vi "RT_stage_control_rev8_loadverification.vi"() -> ()   [LabVIEW 2019]
uses:
  StageControl.ctl
  RasterControl.ctl
  ForceControl.ctl
  <vilib>/Platform/TimedLoop/XDataNode/timing_clust.ctl
  <vilib>/Platform/TimedLoop/XDataNode/nitl_modes.ctl
  <vilib>/Platform/TimedLoop/XDataNode/wakeup.ctl
  <vilib>/FPGAPlugInAG/myRIO-1900/niLvFpga_Open_myRIO-1900.vi
  <vilib>/rvi/interface/common/dynamic/niFpgaDynamicAddResources.vi
  <vilib>/Utility/error.llb/Error Cluster From Error Code.vi
  <vilib>/rvi/errors/niLvFpgaAdjustHostInterfaceError.vi
  <vilib>/FPGAPlugInAG/Dynamic/niLvFpga_Close_Dynamic.vi
  <vilib>/rvi/interface/nirviOpenFPGA/nirviOpenFPGA.xnode
  FPGA Bitfiles/studentchallenge_FPGATarget_FPGARADCWDAC3_YedoVmsa1Hg.lvbitx
  FPGA_2R_ADC_W_DAC.vi
  <vilib>/Platform/TimedLoop/XDataNode/XDataNode.xnode
  <vilib>/rvi/interface/nirviReadWriteControl/nirviReadWriteControl.xnode
  <vilib>/rvi/interface/nirviCloseFPGA/nirviCloseFPGA.xnode
  <vilib>/Platform/TimedLoop/XDataNode/XDNodeRunTimeDep.lvlib
  NiFpgaLv.dll
  <vilib>/rvi/interface/Simulation/niFpgaSimulationCallBeginRW.vi
panel:
  out "load cell out":dbl(graph)
  out "Force Loop":T1
  out "Force Control Late":i16
  in  "Y Manual [mm]":dbl format="%.4f"
  in  "X Manual [mm]":dbl format="%.4f"
  in  "Zero Cap":bool
  in  "Zero Y":bool
  in  "Zero X":bool
  in  "Des Force [N]":dbl=0.3 format="%.3f"
  in  "Return Speed":dbl=5.0 format="%#_13g"
  in  "Step Size [mm]":dbl=0.02 format="%.3f"
  in  "Width [mm]":dbl=3.0 format="%.3f"
  in  "Velocity [mm/s]":dbl=0.1 format="%.3f"
  in  "Stroke [mm]":dbl=3.0 format="%.3f"
  out "Current [A]":dbl=-0.00198361231060317 format="%.4f"
  out "Cap Probe [mm]":dbl=0.43435006179715263 format="%.4f"
  out "X Position [mm]":dbl format="%.4f"
  out "Y Position [mm]":dbl=0.0003125 format="%.4f"
  out "Stage Motion Late":i16
  in  "Start":bool
  in  "Operation":T2=enum."Raster"
  out "Raster Loop":T3
  out "Outer Loop":T2
  in  "stop":bool
  out "settle start":u32
  out "stroke finished":bool=TRUE
  out "ToolDownStart":bool
  out "Tool Up Finished":bool
  out "Tool Down Finished":bool
  out "FPGA Ref":refnum<k20>
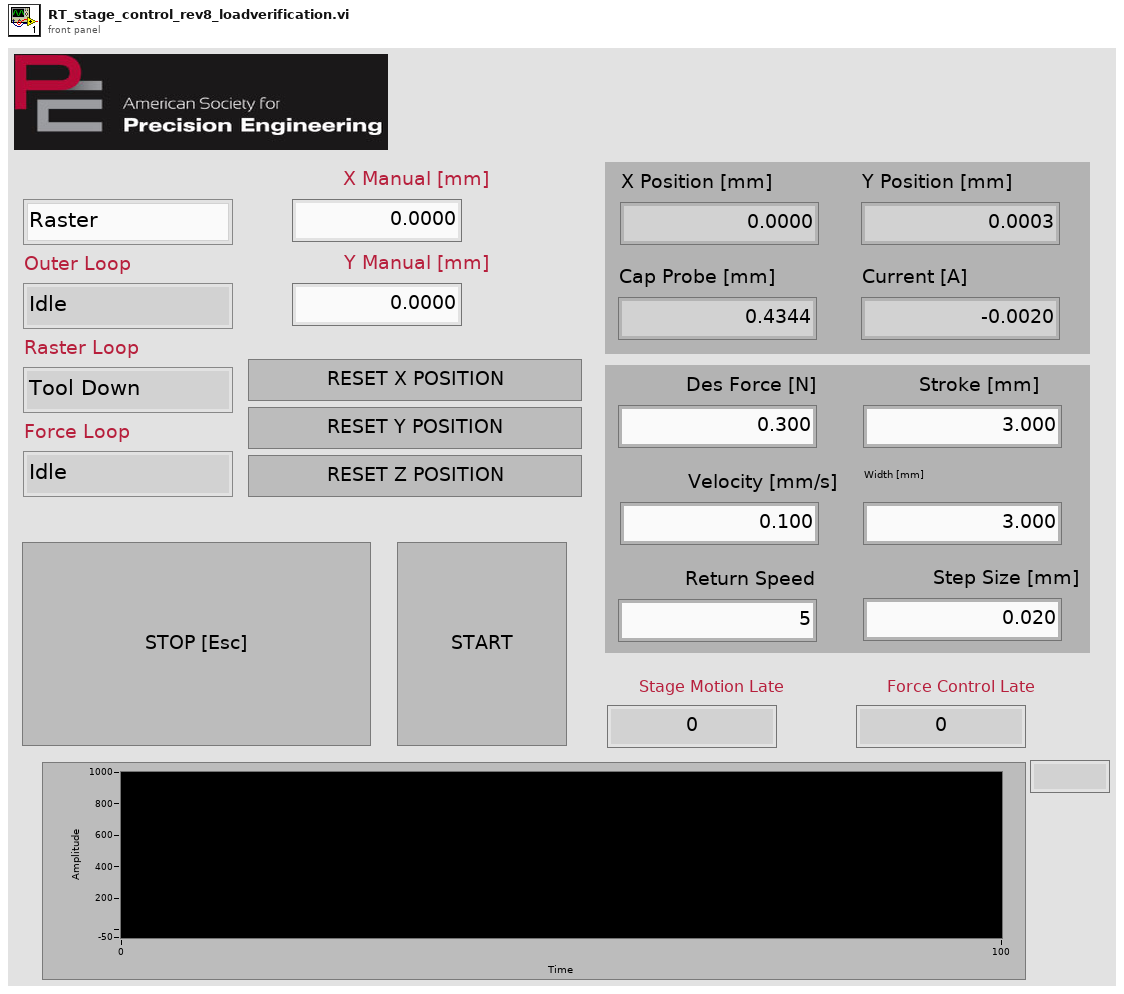
[diagram p1: front panel]
types:
  T1 = typedef "ForceControl.ctl" = enum16{"Idle", "Tool Down", "Force Control", "Tool Up"}
  T2 = typedef "StageControl.ctl" = enum16{"Idle", "Raster", "Home X", "Home Y"}
  T3 = typedef "RasterControl.ctl" = enum16{"Tool Down", "Stroke", "Tool Up", "Return & Step", "Settle", "Return to Zero"}
  T4 = cluster{"Encoder A":i32, "Encoder B":i32, "X Desired [mm]":dbl, "X Position [mm]":dbl, "Y Desired [mm]":dbl, "Y Position [mm]":dbl}
  T5 = typedef "XDNodeRunTimeDep.lvlib/timing_clust.ctl" = cluster{"Expected End [f-1]":u64, "Actual End [f-1]":u64, "Finished Late? [f-1]":bool, "Expected End [i-1]":u64, "Actual End [i-1]":u64, "Finished Late? [i-1]":bool, "Expected Start [i]":u64, "Actual Start [i]":u64, "Expected Start [f]":u64, "Actual Start [f]":u64, "Source Name":string, "Structure Name":string, "Period":i64, "Deadline":i64, "Offset":i64, "Start":i64, "Priority":i32, "Timeout":i32, "Mode":T6, "Wakeup Reason":T7, "Error":errorcluster, "Source Type":string, "Secondary Source Type":string, "Global End Time":u64, "Global Start Time":u64, "Frame Duration":u64, "Iteration Duration":u64, "Assigned CPU":i32, "I/O Scan Engine Mode":u32}
  T6 = typedef "XDNodeRunTimeDep.lvlib/nitl_modes.ctl" = enum32{"No Change", "Process missed periods, maintain original phase", "Discard missed periods, maintain original phase", "Process missed periods, ignore original phase", "Discard missed periods, ignore original phase"}
  T7 = typedef "XDNodeRunTimeDep.lvlib/wakeup.ctl" = enum32{"Normal", "Aborted", "Asynchronous wakeup", "Timing source error", "Timed loop error", "Timeout"}
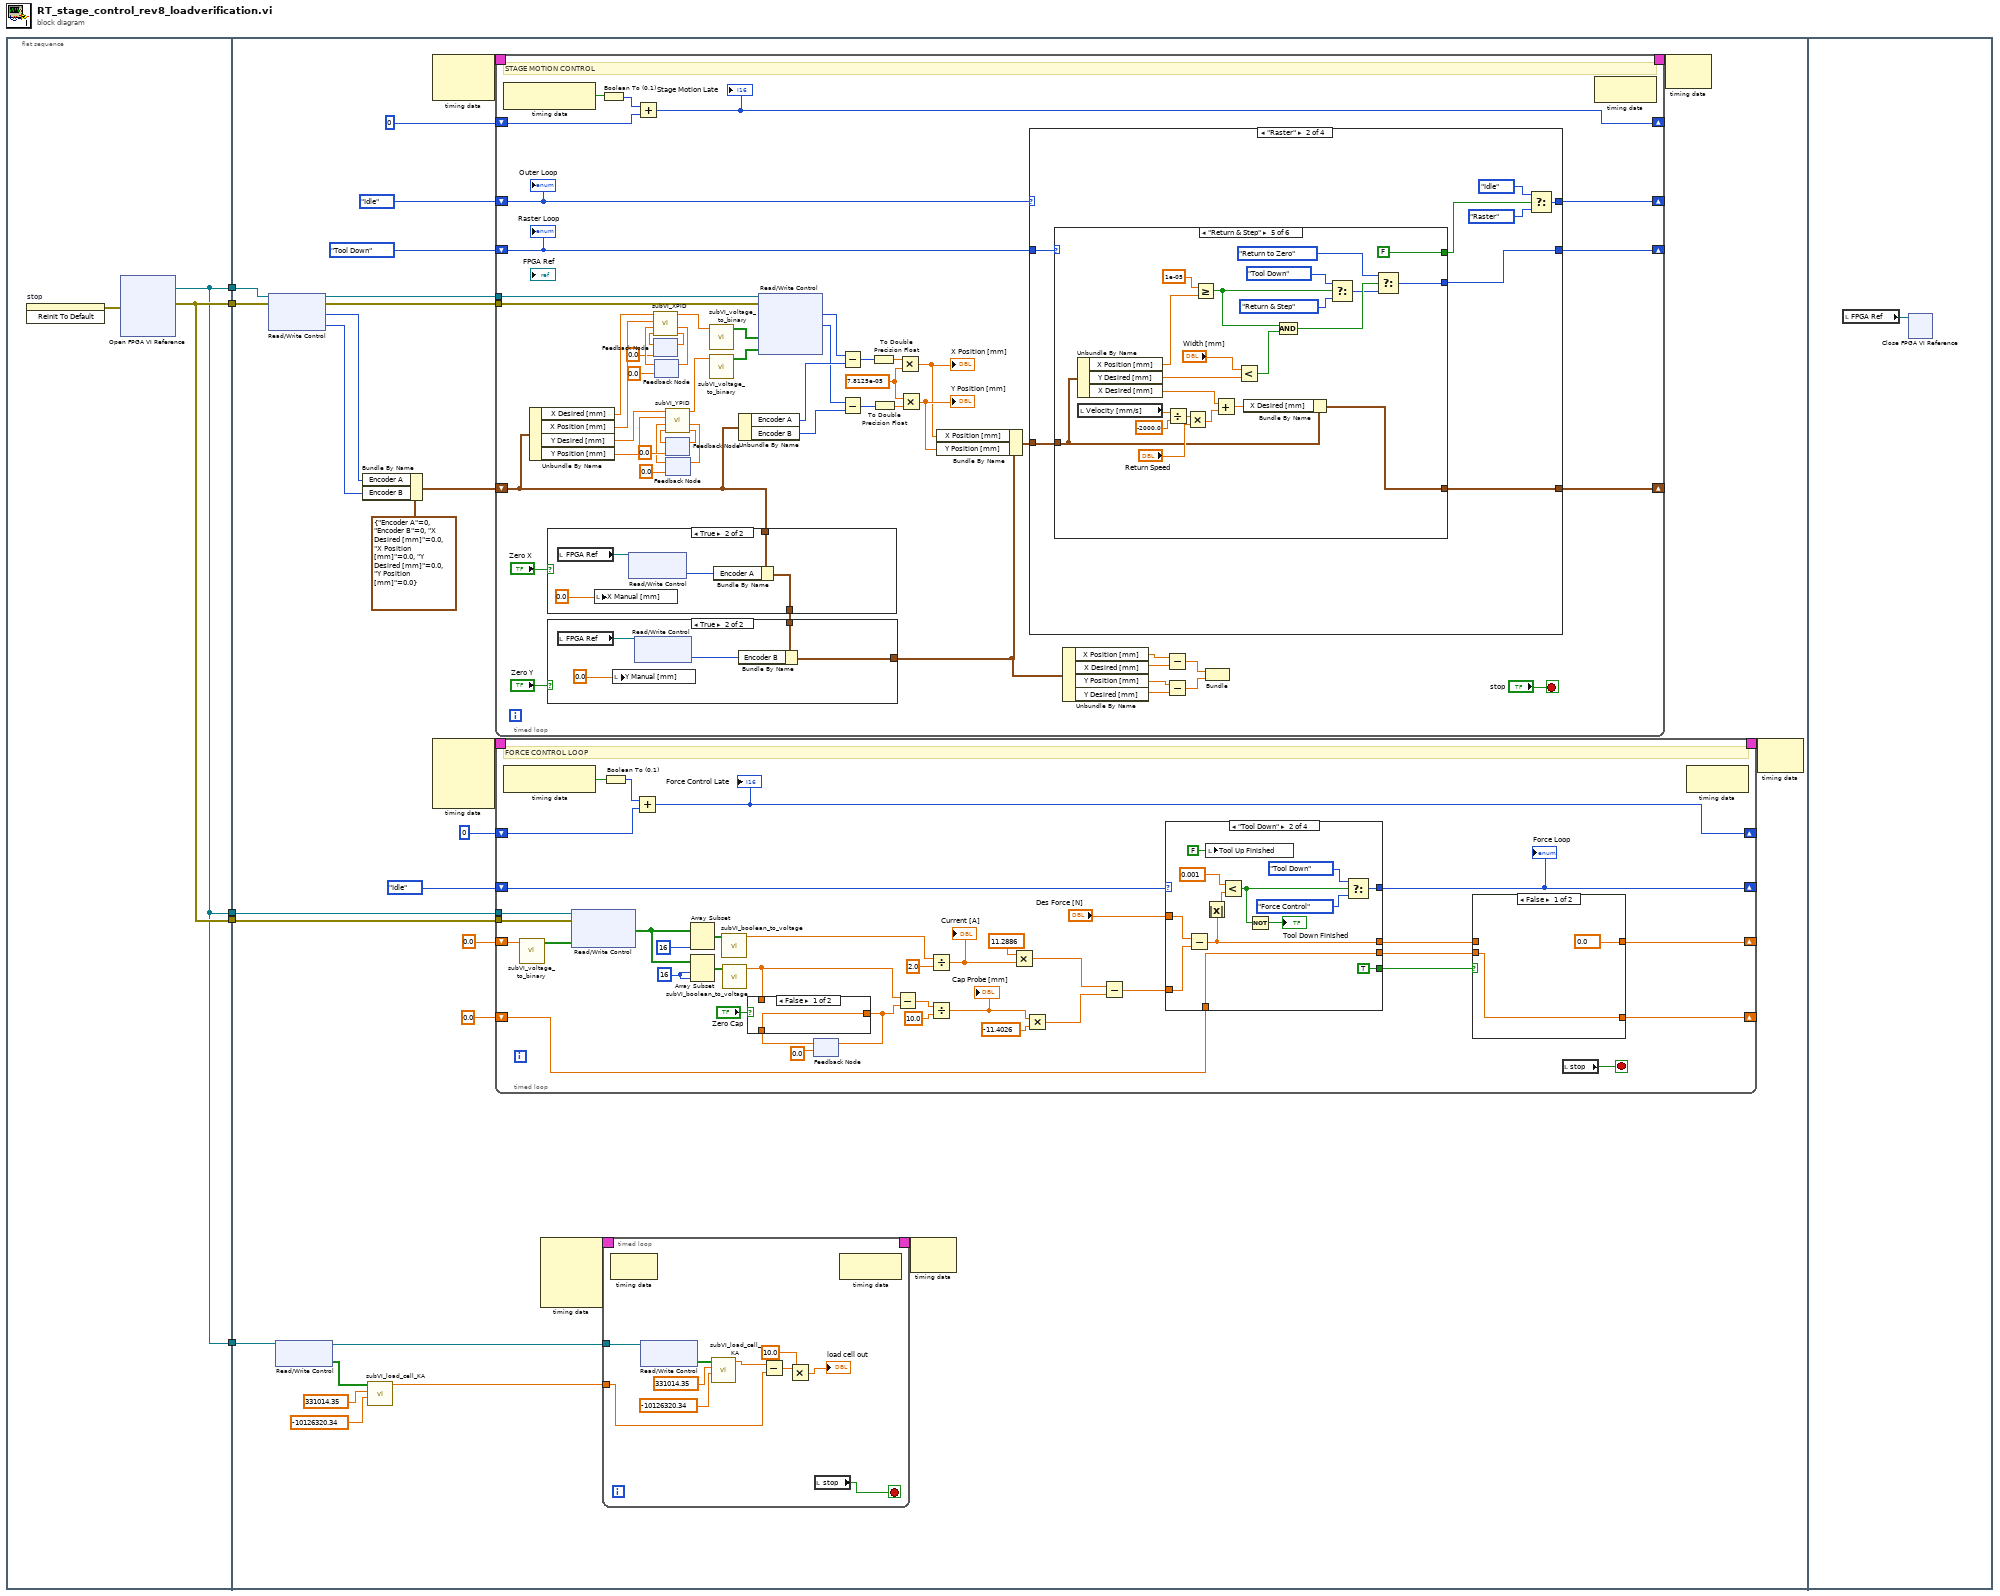
[diagram p0: block diagram]
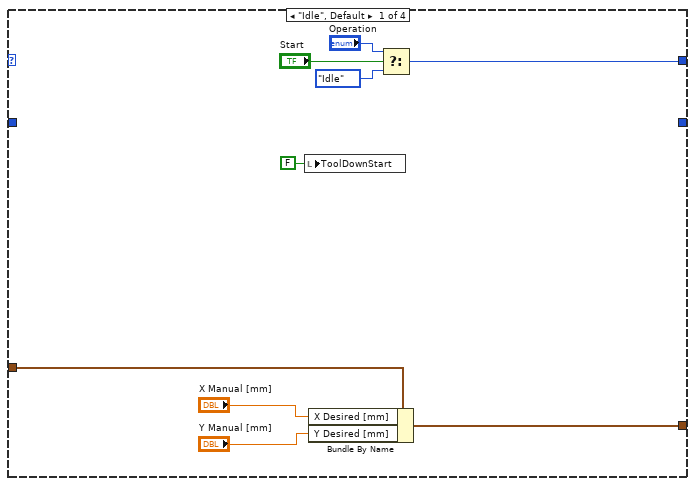
[diagram p2: hidden frame]
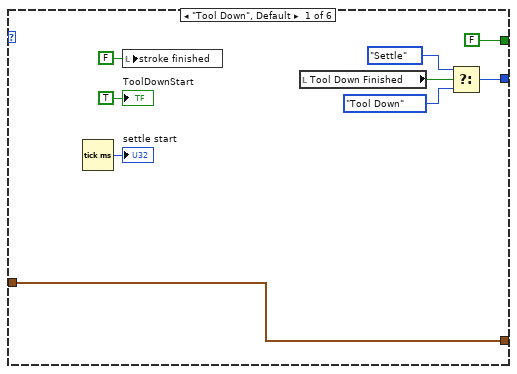
[diagram p3: hidden frame]
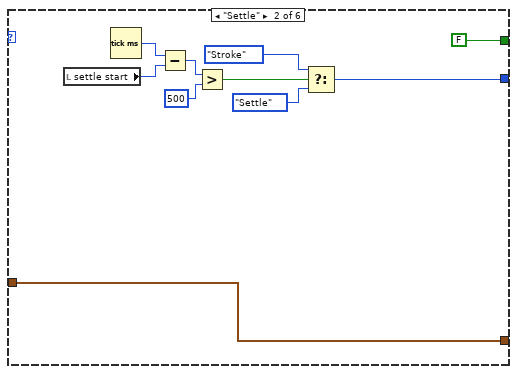
[diagram p4: hidden frame]
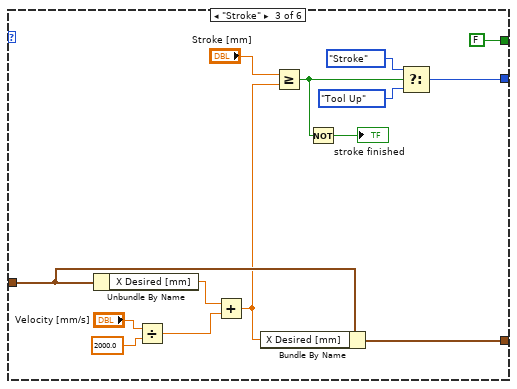
[diagram p5: hidden frame]
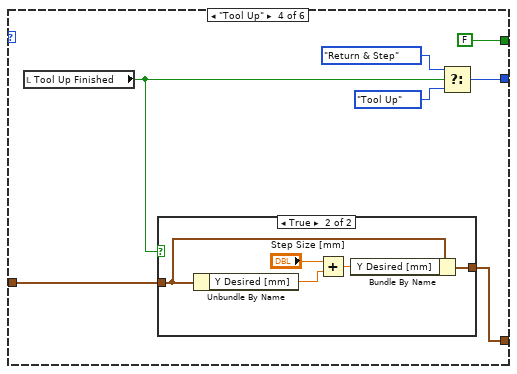
[diagram p6: hidden frame]
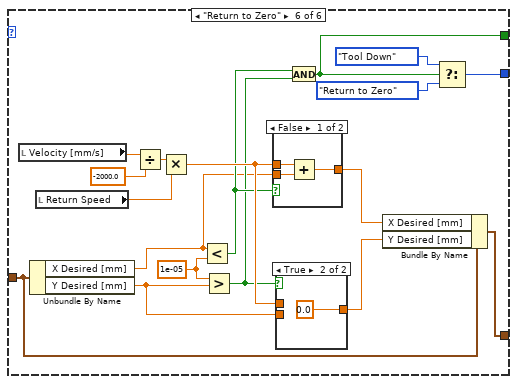
[diagram p8: hidden frame]
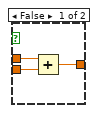
[diagram p9: hidden frame]
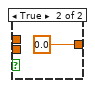
[diagram p10: hidden frame]
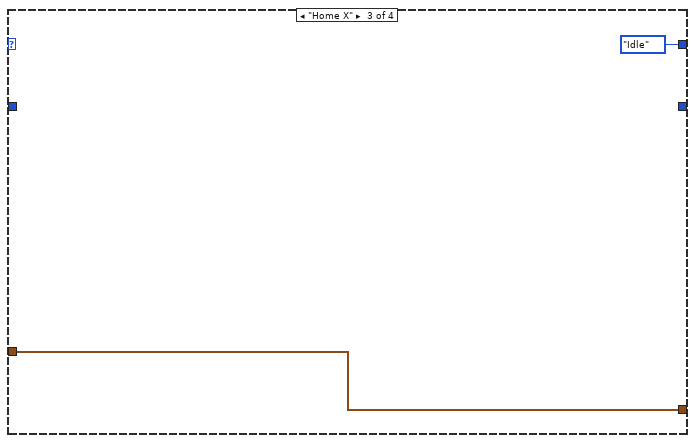
[diagram p11: hidden frame]
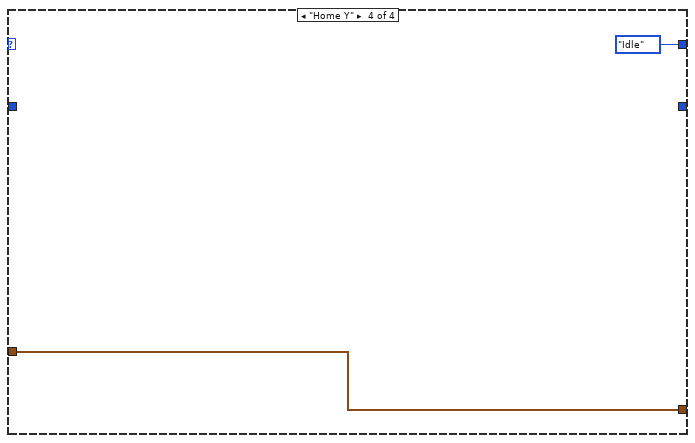
[diagram p12: hidden frame]
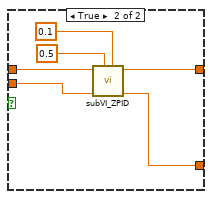
[diagram p15: hidden frame]
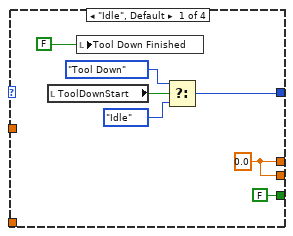
[diagram p17: hidden frame]
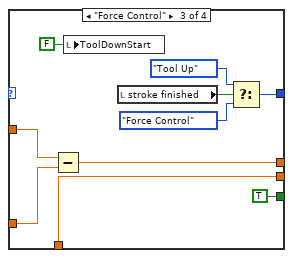
[diagram p18: hidden frame]
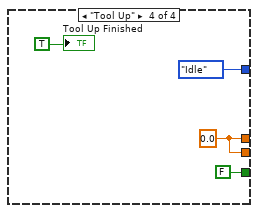
[diagram p19: hidden frame]
diagram:
  n1 = flat-sequence {
    tunnel: [w7] -> w5
    tunnel: [w6] -> w4
    tunnel: [w6] -> w3
    tunnel: [w7] -> w2
    tunnel: [w6] -> w1
    tunnel: w5 -> [w28]
    tunnel: w4 -> [w26]
    tunnel: w3 -> [w15]
    tunnel: w2 -> [w25]
    tunnel: w1 -> [w14]
    frame #0 {
      n2 = invoke on="stop" class="Bool (strict)" method="Reinit To Default"() -> (error out=w8:errorcluster)  [unwired: 3 in, 2 out]
      n3 = xnode "Open FPGA VI Reference"("error in"=w8) -> ("FPGA VI Reference Out"=w6:refnum<k20>, "error out"=w7:errorcluster)  [unwired: 1 in]
    }
    frame #1 {
      n4 = xnode "Read/Write Control"("FPGA VI Reference In"=w26, "error in"=w28) -> ("FPGA VI Reference Out"=w33:refnum<k20>, "error out"=w32:errorcluster, "Encoder A"=w21:i32, "Encoder B"=w22:i32)
      n5 = xnode "Read/Write Control"("FPGA VI Reference In"=w14) -> ("FPGA VI Reference Out"=w13:refnum<k20>, "Data array"=w12:bool[])  [unwired: 1 in, 1 out]
      n6 = Bundle By Name(cluster=T4 {"Encoder A"=0, "Encoder B"=0, "X Desired [mm]"=0.0, "X Position [mm]"=0.0, "Y Desired [mm]"=0.0, "Y Position [mm]"=0.0}, "Encoder A"=w21, "Encoder B"=w22) -> (w23:T4)
      n7 = call "subVI_load_cell_KA.vi"("offset"=-10126320.34, "scale"=331014.35, "DATA ARRAY IN"=w12) -> ("LOAD OUT"=w9:dbl)  [unwired: 8 in]
      n8 = node-c288() -> (w37:T5)  [unwired: 2 in]
      n9 = node-c288() -> (w35:T5)  [unwired: 4 in]
      n10 = timed-loop {
        timing: w37 -> [_]
        timing-out: [_] -> w36
        tunnel: w33 -> [w52]
        tunnel: w32 -> [w105]
        shift-right: [w99] -> _
        shift-left: StageControl."Idle" ("Enum 2") -> [w98]
        shift-right: [w96] -> _
        shift-left: RasterControl."Tool Down" -> [w97]
        shift-right: [w90] -> _
        shift-left: i16 0 -> [w91]
        shift-right: [w72] -> _
        shift-left: w23 -> [w67]
        stop <- "stop" stop-if-true
        w100 = 7.8125e-05 ("y")
        # "STAGE MOTION CONTROL"
        n11 = node-c288() -> (w93:bool)  [unwired: 1 in]
        n12 = Unbundle By Name(w67) -> ("X Desired [mm]"=w71:dbl, "X Position [mm]"=w70:dbl, "Y Desired [mm]"=w69:dbl, "Y Position [mm]"=w68:dbl)
        n13 = case shown="True" "Zero X" {
          tunnel: [w231 w233] -> w73
          tunnel: w67 -> [w231 w232]
          frame False {
          }
          frame True {
            n14 = local read "FPGA Ref"() -> (w235:refnum<k20>)
            n15 = local write "X Manual [mm]"(0.0 ("X Relative Position [mm]")) -> ()
            n16 = xnode "Read/Write Control"("FPGA VI Reference In"=w235) -> ("Encoder A"=w234:i32)  [unwired: 1 in, 2 out]
            n17 = Bundle By Name(cluster=w232, "Encoder A"=w234) -> (w233:T4)
          }
        }
        n18 = case shown="True" "Zero Y" {
          tunnel: w73 -> [w225 w229]
          tunnel: [w225 w226] -> w53
          frame False {
          }
          frame True {
            n19 = local read "FPGA Ref"() -> (w230:refnum<k20>)
            n20 = local write "Y Manual [mm]"(0.0 ("Y Relative Position [mm]")) -> ()
            n21 = xnode "Read/Write Control"("FPGA VI Reference In"=w230) -> ("Encoder B"=w228:i32)  [unwired: 1 in, 2 out]
            n22 = Bundle By Name(cluster=w229, "Encoder B"=w228) -> (w226:T4)
          }
        }
        n23 = Boolean To (0,1)(Boolean=w93) -> (0, 1=w92:i16)
        n24 = Add(x=w92, y=w91) -> (x+y=w90:i16)
        "Stage Motion Late" <- w90
        n25 = feedback #1(0.0 ("Cumulative Error Out")) -> (w85:dbl)
        n26 = feedback #2(0.0 ("Error")) -> (w84:dbl)
        n27 = call "subVI_XPID.vi"("Cumulative Error In"=w85, "Previous Error"=w84, "Encoder Position [mm]"=w70, "Desired Position [mm]"=w71) -> ("Cumulative Error Out"=w87:dbl, "Error"=w86:dbl, "Control Signal [V]"=w75:dbl)  [unwired: 5 in]
        n28 = feedback-in #1(w87) -> ()
        n29 = feedback-in #2(w86) -> ()
        n30 = feedback #3(0.0 ("Cumulative Error Out")) -> (w78:dbl)
        n31 = feedback #4(0.0 ("Error")) -> (w79:dbl)
        n32 = call "subVI_YPID.vi"("Cumulative Error In"=w78, "Previous Error"=w79, "Encoder Position [mm]"=w68, "Desired Position [mm]"=w69) -> ("Cumulative Error Out"=w76:dbl, "Error"=w77:dbl, "Control Signal [V]"=w74:dbl)  [unwired: 5 in]
        n33 = feedback-in #3(w76) -> ()
        n34 = feedback-in #4(w77) -> ()
        n35 = call "subVI_voltage_to_binary.vi"("voltage"=w75) -> ("binary"=w89:bool[])  [unwired: 10 in]
        n36 = call "subVI_voltage_to_binary.vi"("voltage"=w74) -> ("binary"=w88:bool[])  [unwired: 10 in]
        n37 = Unbundle By Name(w67) -> ("Encoder A"=w66:i32, "Encoder B"=w65:i32)
        n38 = xnode "Read/Write Control"("FPGA VI Reference In"=w52, "error in"=w105, "DAC 1 write"=w89, "DAC 2 write"=w88) -> ("Encoder A"=w64:i32, "Encoder B"=w63:i32)  [unwired: 2 out]
        n39 = Subtract(x=w64, y=w66) -> (x-y=w103:i32)
        n40 = Subtract(x=w63, y=w65) -> (x-y=w102:i32)
        n41 = To Double Precision Float(number=w103) -> (double precision float=w104:dbl)
        n42 = To Double Precision Float(number=w102) -> (double precision float=w101:dbl)
        n43 = Multiply(x=w104, y=w100) -> (x*y=w60:dbl)
        "X Position [mm]" <- w60
        n44 = Multiply(x=w100, y=w101) -> (x*y=w61:dbl)
        "Y Position [mm]" <- w61
        n45 = Bundle By Name(cluster=w53, "X Position [mm]"=w60, "Y Position [mm]"=w61) -> (w62:T4)
        n46 = case shown="\"Raster\"" w98 {
          tunnel: [w118 w125 StageControl."Idle" ("Enum 2") StageControl."Idle" ("Enum 2")] -> w99
          tunnel: w97 -> [_ w126 _ _]
          tunnel: [_ w121 _ _] -> w96
          tunnel: w62 -> [w110 w120 w221 w223]
          tunnel: [w111 w119 w221 w223] -> w72
          frame "Idle", Default {
            n47 = local write "ToolDownStart"(FALSE ("ToolDownStart")) -> ()
            n48 = Bundle By Name(cluster=w110, "X Desired [mm]"="X Manual [mm]", "Y Desired [mm]"="Y Manual [mm]") -> (w111:T4)
            n49 = Select(t="Operation", s="Start", f=StageControl."Idle" ("Enum 2")) -> (s? t:f=w118:T2)
          }
          frame "Raster" {
            n50 = case shown="\"Return & Step\"" w126 {
              tunnel: [FALSE FALSE FALSE FALSE FALSE w207] -> w122
              tunnel: [w134 w144 w156 w161 w177 w209] -> w121
              tunnel: [w128 w136 w153 w164 w181 w200] -> w119
              tunnel: w120 -> [w128 w136 w150 w160 w173 w197]
              frame "Tool Down", Default {
                n51 = Tick Count (ms)() -> (millisecond timer value=→"settle start":u32)
                n52 = local write "stroke finished"(FALSE ("stroke finished")) -> ()
                n53 = local read "Tool Down Finished"() -> (w131:bool)
                n54 = Select(t=RasterControl."Settle", s=w131, f=RasterControl."Tool Down") -> (s? t:f=w134:T3)
                "ToolDownStart" <- TRUE
              }
              frame "Settle" {
                n55 = local read "settle start"() -> (w137:u32)
                n56 = Tick Count (ms)() -> (millisecond timer value=w142:u32)
                n57 = Subtract(x=w142, y=w137) -> (x-y=w141:u32)
                n58 = Greater?(x=w141, y=u32 500) -> (0:w138:bool)
                n59 = Select(t=RasterControl."Stroke", s=w138, f=RasterControl."Settle") -> (s? t:f=w144:T3)
              }
              frame "Stroke" {
                n60 = Unbundle By Name(w150) -> ("X Desired [mm]"=w149:dbl)
                n61 = Divide(x="Velocity [mm/s]", y=2000.0) -> (x/y=w151:dbl)
                n62 = Add(x=w149, y=w151) -> (x+y=w148:dbl)
                n63 = Bundle By Name(cluster=w150, "X Desired [mm]"=w148) -> (w153:T4)
                n64 = Greater Or Equal?(x="Stroke [mm]", y=w148) -> (x >= y?=w147:bool)
                n65 = Not(x=w147) -> (.not. x?=→"stroke finished":bool)
                n66 = Select(t=RasterControl."Stroke", s=w147, f=RasterControl."Tool Up") -> (s? t:f=w156:T3)
              }
              frame "Tool Up" {
                n67 = local read "Tool Up Finished"() -> (w163:bool)
                n68 = case shown="True" w163 {
                  tunnel: [w167 w171] -> w164
                  tunnel: w160 -> [w167 w168]
                  frame False {
                  }
                  frame True {
                    n69 = Unbundle By Name(w168) -> ("Y Desired [mm]"=w169:dbl)
                    n70 = Add(x="Step Size [mm]", y=w169) -> (x+y=w172:dbl)
                    n71 = Bundle By Name(cluster=w168, "Y Desired [mm]"=w172) -> (w171:T4)
                  }
                }
                n72 = Select(t=RasterControl."Return & Step", s=w163, f=RasterControl."Tool Up") -> (s? t:f=w161:T3)
              }
              frame "Return & Step" {
                n73 = Unbundle By Name(w173) -> ("X Position [mm]"=w175:dbl, "Y Desired [mm]"=w174:dbl, "X Desired [mm]"=w176:dbl)
                n74 = local read "Velocity [mm/s]"() -> (w192:dbl)
                n75 = Divide(x=w192, y=-2000.0) -> (x/y=w190:dbl)
                n76 = Multiply(x=w190, y="Return Speed") -> (x*y=w182:dbl)
                n77 = Greater Or Equal?(x=1e-05 ("y"), y=w175) -> (x >= y?=w184:bool)
                n78 = Add(x=w176, y=w182) -> (x+y=w183:dbl)
                n79 = Less?(x="Width [mm]", y=w174) -> (x < y?=w178:bool)
                n80 = Bundle By Name(cluster=w173, "X Desired [mm]"=w183) -> (w181:T4)
                n81 = And(x=w184, y=w178) -> (x .and. y?=w187:bool)
                n82 = Select(t=RasterControl."Tool Down", s=w184, f=RasterControl."Return & Step") -> (s? t:f=w186:T3)
                n83 = Select(t=RasterControl."Return to Zero", s=w187, f=w186) -> (s? t:f=w177:T3)
              }
              frame "Return to Zero" {
                w204 = 1e-05 ("y")
                n84 = local read "Velocity [mm/s]"() -> (w212:dbl)
                n85 = Unbundle By Name(w197) -> ("X Desired [mm]"=w196:dbl, "Y Desired [mm]"=w195:dbl)
                n86 = local read "Return Speed"() -> (w205:dbl)
                n87 = Divide(x=w212, y=-2000.0) -> (x/y=w210:dbl)
                n88 = Multiply(x=w210, y=w205) -> (x*y=w203:dbl)
                n89 = Less?(x=w196, y=w204) -> (x < y?=w199:bool)
                n90 = Greater?(x=w204, y=w195) -> (0:w198:bool)
                n91 = case shown="False" w199 {
                  tunnel: w203 -> [w219 _]
                  tunnel: [w218 0.0] -> w202
                  tunnel: w196 -> [w217 _]
                  frame False {
                    n92 = Add(x=w219, y=w217) -> (x+y=w218:dbl)
                  }
                  frame True {
                  }
                }
                n93 = case shown="True" w198 {
                  tunnel: w203 -> [w215 _]
                  tunnel: [w214 0.0] -> w201
                  tunnel: w195 -> [w213 _]
                  frame False {
                    n94 = Add(x=w215, y=w213) -> (x+y=w214:dbl)
                  }
                  frame True {
                  }
                }
                n95 = And(x=w199, y=w198) -> (x .and. y?=w207:bool)
                n96 = Bundle By Name(cluster=w197, "X Desired [mm]"=w202, "Y Desired [mm]"=w201) -> (w200:T4)
                n97 = Select(t=RasterControl."Tool Down", s=w207, f=RasterControl."Return to Zero") -> (s? t:f=w209:T3)
              }
            }
            n98 = Select(t=StageControl."Idle" ("Enum 2"), s=w122, f=StageControl."Raster" ("Enum 2")) -> (s? t:f=w125:T2)
          }
          frame "Home X" {
          }
          frame "Home Y" {
          }
        }
        n99 = Unbundle By Name(w53) -> ("X Position [mm]"=w56:dbl, "X Desired [mm]"=w57:dbl, "Y Position [mm]"=w58:dbl, "Y Desired [mm]"=w59:dbl)
        n100 = Subtract(x=w56, y=w57) -> (x-y=w55:dbl)
        n101 = Subtract(x=w58, y=w59) -> (x-y=w54:dbl)
        n102 = Bundle(w55, w54) -> ()  [unwired: 1 in, 1 out]
        n103 = node-c288() -> ()  [unwired: 1 in, 1 out]
        "Outer Loop" <- w98
        "Raster Loop" <- w97
      }
      n104 = timed-loop {
        timing: w35 -> [_]
        timing-out: [_] -> w34
        shift-right: [w238] -> _
        shift-left: ForceControl."Idle" -> [w267]
        tunnel: w15 -> [w257]
        tunnel: w25 -> [w256]
        shift-right: [w239] -> _
        shift-left: 0.0 -> [w253]
        shift-right: [w247] -> _
        shift-left: 0.0 ("Cumulative Error Out") -> [w245]
        shift-right: [w241] -> _
        shift-left: i16 0 -> [w244]
        stop <- w276 stop-if-true
        w274 = 16 ("length")
        # "FORCE CONTROL LOOP"
        n105 = node-c288() -> (w243:bool)  [unwired: 1 in]
        n106 = call "subVI_voltage_to_binary.vi"("voltage"=w253) -> ("binary"=w254:bool[])  [unwired: 10 in]
        n107 = xnode "Read/Write Control"("FPGA VI Reference In"=w257, "error in"=w256, "DAC 3 write"=w254) -> ("ADC Read"=w266:bool[])  [unwired: 2 out]
        n108 = Boolean To (0,1)(Boolean=w243) -> (0, 1=w242:i16)
        n109 = Add(x=w242, y=w244) -> (x+y=w241:i16)
        "Force Control Late" <- w241
        n110 = Array Subset(array=w266, length=16) -> (w275:bool[])  [unwired: 1 in]
        n111 = Array Subset(array=w266, index=w274, length=w274) -> (w273:bool[])
        n112 = call "subVI_boolean_to_voltage.vi"("ADC read"=w275) -> ("V"=w248:dbl)  [unwired: 10 in]
        n113 = call "subVI_boolean_to_voltage.vi"("ADC read"=w273) -> ("V"=w260:dbl)  [unwired: 10 in]
        n114 = feedback #5(0.0) -> (w259:dbl)
        n115 = case shown="False" "Zero Cap" {
          tunnel: [w285 w286] -> w255
          tunnel: w259 -> [w285 _]
          tunnel: w260 -> [_ w286]
          frame False {
          }
          frame True {
          }
        }
        n116 = feedback-in #5(w255) -> ()
        n117 = Subtract(x=w260, y=w255) -> (x-y=w263:dbl)
        n118 = Divide(x=w248, y=2.0) -> (x/y=w268:dbl)
        "Current [A]" <- w268
        n119 = Divide(x=w263, y=10.0) -> (x/y=w258:dbl)
        "Cap Probe [mm]" <- w258
        n120 = Multiply(x=11.2886 ("BL"), y=w268) -> (x*y=w265:dbl)
        n121 = Multiply(x=w258, y=-11.4026 ("Stiffness [N/m]")) -> (x*y=w264:dbl)
        n122 = Subtract(x=w265, y=w264) -> (x-y=w249:dbl)
        n123 = case shown="\"Tool Down\"" w267 {
          tunnel: [w290 w304 w316 ForceControl."Idle"] -> w238
          tunnel: "Des Force [N]" -> [_ w302 w310 _]
          tunnel: w249 -> [_ w301 w309 _]
          tunnel: [w287 w298 w311 w317] -> w251
          tunnel: [FALSE TRUE TRUE FALSE] -> w240
          tunnel: [w287 w294 w307 w317] -> w246
          tunnel: w245 -> [_ w294 w307 _]
          frame "Idle", Default {
            w287 = 0.0
            n124 = local read "ToolDownStart"() -> (w291:bool)
            n125 = local write "Tool Down Finished"(FALSE ("Tool Down Finished")) -> ()
            n126 = Select(t=ForceControl."Tool Down", s=w291, f=ForceControl."Idle") -> (s? t:f=w290:T1)
          }
          frame "Tool Down" {
            n127 = Subtract(x=w302, y=w301) -> (x-y=w298:dbl)
            n128 = Absolute Value(x=w298) -> (abs(x)=w299:dbl)
            n129 = local write "Tool Up Finished"(FALSE ("Tool Up Finished")) -> ()
            n130 = Less?(x=0.001 ("error threshold"), y=w299) -> (x < y?=w296:bool)
            n131 = Not(x=w296) -> (.not. x?=→"Tool Down Finished":bool)
            n132 = Select(t=ForceControl."Tool Down", s=w296, f=ForceControl."Force Control") -> (s? t:f=w304:T1)
          }
          frame "Force Control" {
            n133 = Subtract(x=w310, y=w309) -> (x-y=w311:dbl)
            n134 = local write "ToolDownStart"(FALSE ("ToolDownStart")) -> ()
            n135 = local read "stroke finished"() -> (w315:bool)
            n136 = Select(t=ForceControl."Tool Up", s=w315, f=ForceControl."Force Control") -> (s? t:f=w316:T1)
          }
          frame "Tool Up" {
            w317 = 0.0
            "Tool Up Finished" <- TRUE ("Tool Up Finished")
          }
        }
        "Force Loop" <- w238
        n137 = case shown="False" w240 {
          tunnel: w251 -> [_ w284]
          tunnel: [0.0 ("Z Manual") w283] -> w239
          tunnel: [w277 w280] -> w247
          tunnel: w246 -> [w277 w279]
          frame False {
          }
          frame True {
            n138 = call "subVI_ZPID.vi"("I"=0.1, "P"=0.5, "Cumulative Error In"=w279, "Error In"=w284) -> ("Cumulative Error Out"=w280:dbl, "Control Signal [V]"=w283:dbl)  [unwired: 6 in]
          }
        }
        n139 = local read "stop"() -> (w276:bool)
        n140 = node-c288() -> ()  [unwired: 1 in, 1 out]
      }
      n141 = node-c288() -> (w17:T5)  [unwired: 4 in]
      n142 = timed-loop {
        timing: w17 -> [_]
        timing-out: [_] -> w16
        tunnel: w13 -> [w47]
        tunnel: w9 -> [w42]
        stop <- w38 stop-if-true
        n143 = node-c288() -> ()  [unwired: 1 in, 1 out]
        n144 = xnode "Read/Write Control"("FPGA VI Reference In"=w47) -> ("Data array"=w46:bool[])  [unwired: 1 in, 2 out]
        n145 = call "subVI_load_cell_KA.vi"("offset"=-10126320.34, "scale"=331014.35, "DATA ARRAY IN"=w46) -> ("LOAD OUT"=w43:dbl)  [unwired: 8 in]
        n146 = Subtract(x=w43, y=w42) -> (x-y=w41:dbl)
        n147 = Multiply(x=w41, y=10.0) -> (x*y=→"load cell out":dbl)
        n148 = local read "stop"() -> (w38:bool)
        n149 = node-c288() -> ()  [unwired: 1 in, 1 out]
      }
      n150 = node-c288(w16) -> ()  [unwired: 1 out]
      n151 = node-c288(w36) -> ()  [unwired: 1 out]
      n152 = node-c288(w34) -> ()  [unwired: 1 out]
    }
    frame #2 {
      n153 = local read "FPGA Ref"() -> (w327:refnum<k20>)
      n154 = xnode "Close FPGA VI Reference"("FPGA VI Reference In"=w327) -> ()  [unwired: 1 in, 1 out]
    }
  }
